vi "GCM CCM additional authenticated data.vi"(8 "error in":errorcluster, 10 "data in":string, 11 "lvlibcrypto digest in":refnum<class "lvlibcrypto cipher.lvclass">) -> (0 "error out":errorcluster, 3 "lvlibcrypto digest out":refnum<class "lvlibcrypto cipher.lvclass">)   [LabVIEW 2016, in "lvlibcrypto cipher.lvclass"]
uses:
  lvlibcrypto cipher.lvclass
  lvlibcrypto cipher.lvclass/lvlibcrypto cipher.ctl
  lv tls dll.lvlib
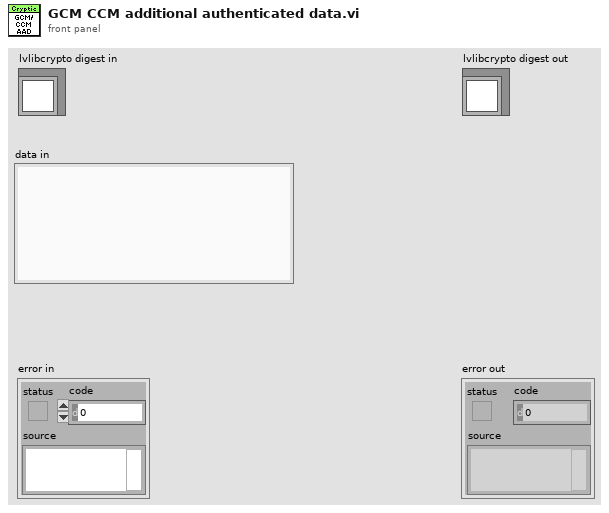
[diagram p1: front panel]
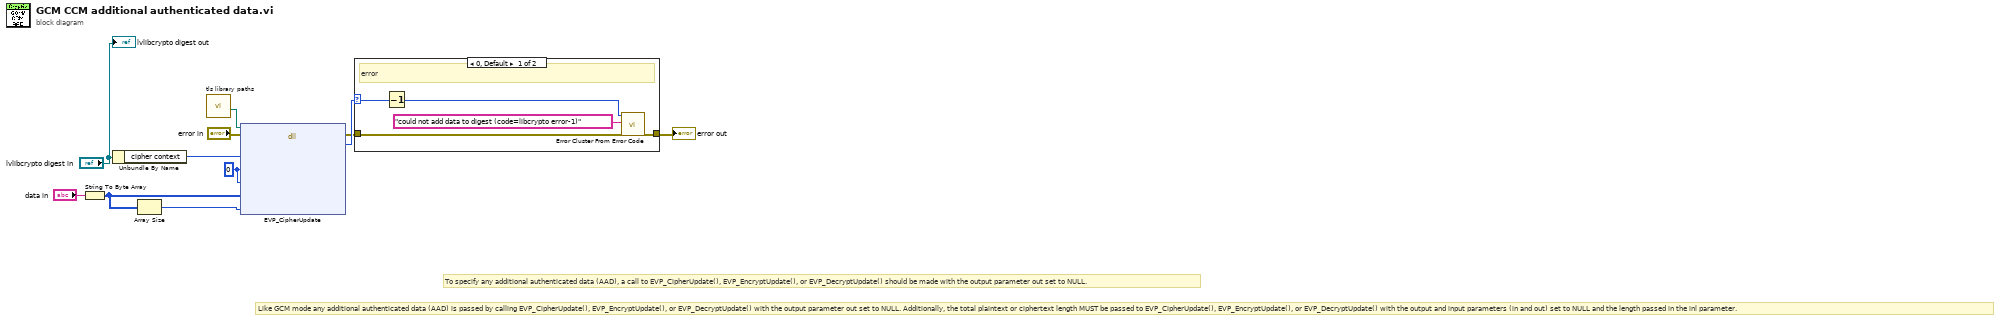
[diagram p0: block diagram]
diagram:
  w1 = u64 0 ("out")
  # "Like GCM mode any additional authenticated data (AAD) is passed by calling EVP_CipherUpdate(), EVP_EncryptUpdate(), or EVP_DecryptUpdate() with the output parameter out set to NULL. Additionally, the total plaintext or ciphertext length MUST be passed to EVP_CipherUpdate(), EVP_EncryptUpdate(), or EVP_DecryptUpdate() with the output and input parameters (in and out) set to NULL and the length passed in the inl parameter."
  # "To specify any additional authenticated data (AAD), a call to EVP_CipherUpdate(), EVP_EncryptUpdate(), or EVP_DecryptUpdate() should be made with the output parameter out set to NULL."
  n1 = String To Byte Array(string="data in") -> (unsigned byte array=w3:u8[])
  n2 = Unbundle By Name("lvlibcrypto digest in") -> ("cipher context"=w5:u64)
  n3 = Array Size(array=w3) -> (size(s)=w2:i32)
  n4 = call "tls library paths.vi"() -> ("libcrypto"=w10:path)  [unwired: 8 in, 3 out]
  n5 = dll-call lib="C:/Users/IEUser/Desktop/tlssimple/libcrypto-41.dll" fn="EVP_CipherUpdate"(path in=w10, error in="error in", "context"=w5, "out"=w1, "outlength"=w1, "in"=w3, "inlength"=w2) -> (error out=w6:errorcluster, "ret"=w7:i32)  [unwired: 6 in, 1 out]
  n6 = case shown="0, Default" w7 {
    selector: w7 -> [w14 _]
    tunnel: [w15 w17] -> w9
    tunnel: w6 -> [w16 w17]
    frame 0, Default {
      # "error"
      n7 = Decrement(x=w14) -> (x-1=w13:i32)
      n8 = call <vilib>:"Error Cluster From Error Code.vi"("error in (no error)"=w16, "error message (\"\")"="could not add data to digest (code=libcrypto error-1)" ("error message (\"\")"), "error code (0)"=w13) -> ("error out"=w15:errorcluster)  [unwired: 6 in]
    }
    frame 1 {
      # "success"
    }
  }
  "error out" <- w9
  "lvlibcrypto digest out" <- "lvlibcrypto digest in"
